vi "Read start.vi"(8 "error in (no error)":errorcluster, 11 "Plot_waveform in":refnum<class "Plot_waveform.lvclass">) -> (0 "error out":errorcluster, 2 "start":timestamp, 3 "Plot_waveform out":refnum<class "Plot_waveform.lvclass">)   [LabVIEW 2019, in "Plot_waveform.lvclass"]
uses:
  Plot_waveform.lvclass
  Plot_waveform.lvclass/Plot_waveform.ctl
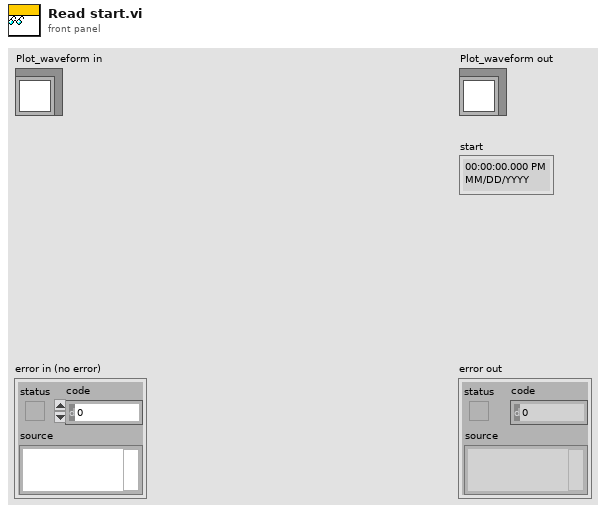
[diagram p1: front panel]
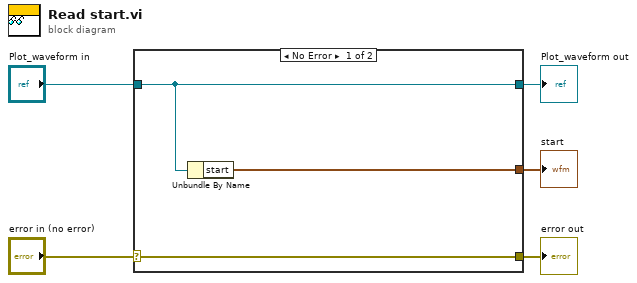
[diagram p0: block diagram]
diagram:
  n1 = case shown="No Error" "error in (no error)" {
    selector: "error in (no error)" -> [w8 w9]
    tunnel: [w8 w9] -> w4
    tunnel: [w7 w10] -> w2
    tunnel: "Plot_waveform in" -> [w7 w10]
    tunnel: [w6 _] -> w1
    frame No Error {
      n2 = Unbundle By Name(w7) -> ("start"=w6:timestamp)
    }
    frame Error {
    }
  }
  "error out" <- w4
  "Plot_waveform out" <- w2
  "start" <- w1
